vi "Get ECAT File Paths.vi"(8 "error in":errorcluster, 11 "ECAT File":T1) -> (0 "error out":errorcluster, 3 "File Path":path)   [LabVIEW 2019, in "SEECD System Explorer.lvlib"]
uses:
  SEECD System Explorer.lvlib
  ECAT Files.ctl
  <vilib>/registry/registry.llb/Registry RtKey.ctl
  <vilib>/registry/registry.llb/Registry SAM.ctl
  <vilib>/registry/registry.llb/Read Registry Value Simple STR.vi
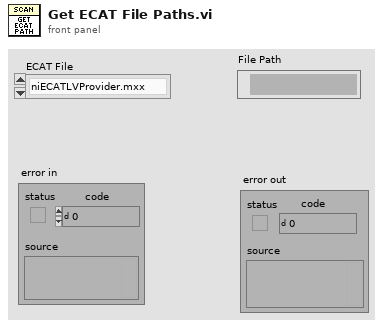
[diagram p1: front panel]
types:
  T1 = typedef "SEECD System Explorer.lvlib/ECAT Files.ctl" = enum16{"niECATLVProvider.mxx", "indcomecat.chm", "Providers DD", "Shared DD"}
  T2 = typedef "Registry SAM.ctl" = enum32{"KEY_QUERY_VALUE", "KEY_SET_VALUE", "KEY_CREATE_SUB_KEY", "KEY_ENUMERATE_SUB_KEYS", "KEY_NOTIFY", "KEY_CREATE_LINK", "KEY_READ", "KEY_WRITE", "KEY_ALL_ACCESS", "KEY_READ | KEY_WRITE"}
  T3 = typedef "Registry RtKey.ctl" = enum32{"HKEY_CLASSES_ROOT", "HKEY_CURRENT_USER", "HKEY_LOCAL_MACHINE", "HKEY_USERS", "HKEY_PERFORMANCE_DATA", "HKEY_CURRENT_CONFIG", "HKEY_DYN_DATA"}
  T4 = typedef "Registry refnum.ctl" = refnum<k1>
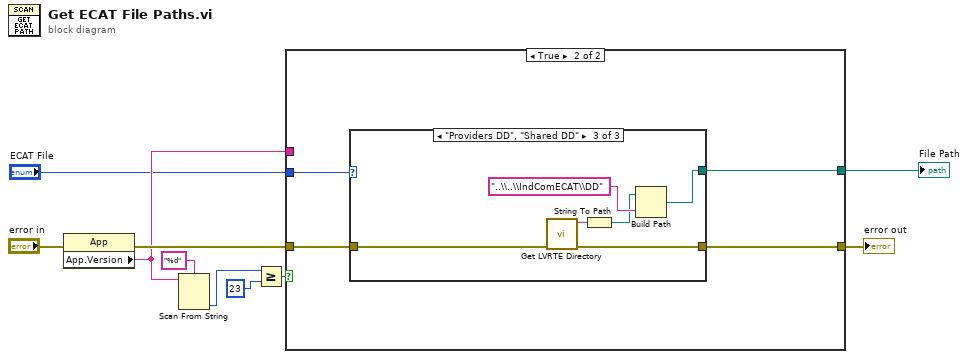
[diagram p0: block diagram]
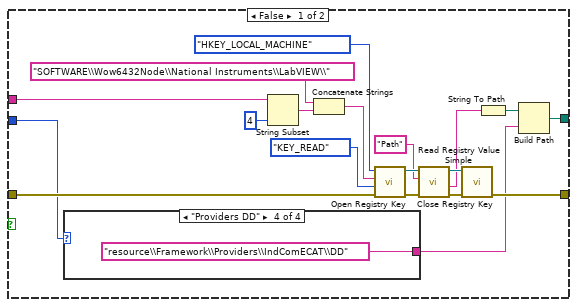
[diagram p2: hidden frame]
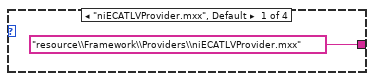
[diagram p3: hidden frame]
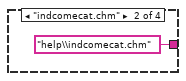
[diagram p4: hidden frame]
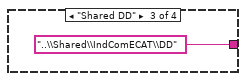
[diagram p5: hidden frame]
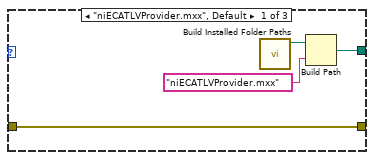
[diagram p6: hidden frame]
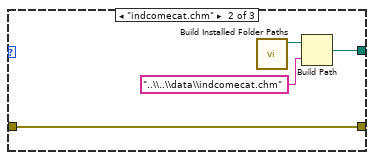
[diagram p7: hidden frame]
diagram:
  n1 = property class="App"(error in="error in") -> (error out=w8:errorcluster, "App.Version"=w4:string)  [unwired: 1 in, 1 out]
  n2 = Scan From String(format string="%d", input string=w4) -> (output 1=w5:i32)  [unwired: 3 in, 3 out]
  n3 = Greater Or Equal?(x=w5, y=23) -> (x >= y?=w3:bool)
  n4 = case shown="True" w3 {
    tunnel: [w23 w34] -> w10
    tunnel: w8 -> [w17 w37]
    tunnel: w4 -> [w15 _]
    tunnel: [w13 w35] -> w2
    tunnel: "ECAT File" -> [w12 w36]
    frame False {
      n5 = case shown="\"Providers DD\"" w12 {
        tunnel: ["resource\\Framework\\Providers\\niECATLVProvider.mxx" "help\\indcomecat.chm" ("name or relative path") "..\\Shared\\IndComECAT\\DD" ("name or relative path") "resource\\Framework\\Providers\\IndComECAT\\DD" ("name or relative path")] -> w11
        frame "niECATLVProvider.mxx", Default {
        }
        frame "indcomecat.chm" {
        }
        frame "Shared DD" {
        }
        frame "Providers DD" {
        }
      }
      n6 = String Subset(string=w15, length (rest)=4 ("length (rest)")) -> (substring=w19:string)  [unwired: 1 in]
      n7 = Concatenate Strings("SOFTWARE\\Wow6432Node\\National Instruments\\LabVIEW\\", w19) -> (w18:string)
      n8 = call <vilib>:"Open Registry Key.vi"("error in (no error)"=w17, "security access mask (KEY_READ | KEY_WRITE)"=Registry_SAM."KEY_READ", "subkey"=w18, "root key (HKEY_LOCAL_MACHINE)"=Registry_RtKey."HKEY_LOCAL_MACHINE") -> ("error out"=w25:errorcluster, "refnum out"=w24:T4)  [unwired: 6 in]
      n9 = call-poly <vilib>:"Read Registry Value Simple.vi"("error in (no error)"=w25, "value"="Path", "refnum"=w24) -> ("error out"=w29:errorcluster, "String/Binary data"=w16:string, "refnum out"=w28:T4)  [unwired: 3 in, 1 out]
      n10 = call <vilib>:"Close Registry Key.vi"("error in (no error)"=w29, "refnum"=w28) -> ("error out"=w23:errorcluster)  [unwired: 5 in]
      n11 = String To Path(string=w16) -> (path=w14:path)
      n12 = Build Path(base path=w14, name or relative path=w11) -> (appended path=w13:path)
    }
    frame True {
      n13 = case shown="\"Providers DD\", \"Shared DD\"" w36 {
        tunnel: w37 -> [w41 w43 w50]
        tunnel: [w39 w45 w46] -> w35
        tunnel: [w41 w43 w49] -> w34
        frame "niECATLVProvider.mxx", Default {
          n14 = call "Build Installed Folder Paths.vi"() -> ("Data Folder Path"=w38:path)  [unwired: 10 in, 1 out]
          n15 = Build Path(base path=w38, name or relative path="niECATLVProvider.mxx") -> (appended path=w39:path)
        }
        frame "indcomecat.chm" {
          n16 = call "Build Installed Folder Paths.vi"() -> ("Data Folder Path"=w42:path)  [unwired: 10 in, 1 out]
          n17 = Build Path(base path=w42, name or relative path="..\\..\\data\\indcomecat.chm") -> (appended path=w45:path)
        }
        frame "Providers DD", "Shared DD" {
          n18 = call "Get LVRTE Directory.vi"("error in"=w50) -> ("error out"=w49:errorcluster, "LVRTE 2022 Directory"=w51:string)  [unwired: 9 in]
          n19 = String To Path(string=w51) -> (path=w47:path)
          n20 = Build Path(base path=w47, name or relative path="..\\..\\IndComECAT\\DD") -> (appended path=w46:path)
        }
      }
    }
  }
  "error out" <- w10
  "File Path" <- w2
